vi "Get Classes to Inherit From.vi"(8 "error in (no error)":errorcluster, 11 "New Class Dialog In":refnum<class "New Class Dialog.lvclass">) -> (0 "error out":errorcluster, 3 "New Class Dialog Out":refnum<class "New Class Dialog.lvclass">)   [LabVIEW 2020, in "Process Generation.lvlib" / "New Class Dialog.lvclass"]
uses:
  New Class Dialog.lvclass
  Framework/Process/Process.lvclass
  Framework/Application/Application.lvclass
  C:/Users/anton/Documents/GitHub/Triarc-Framework/source/Framework/Process/Process.lvclass
  Framework/View/View.lvclass
  New Class Dialog.lvclass/New Class Dialog.ctl
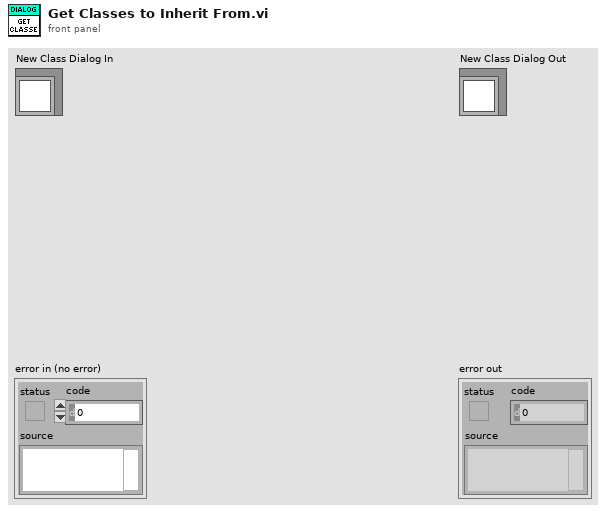
[diagram p1: front panel]
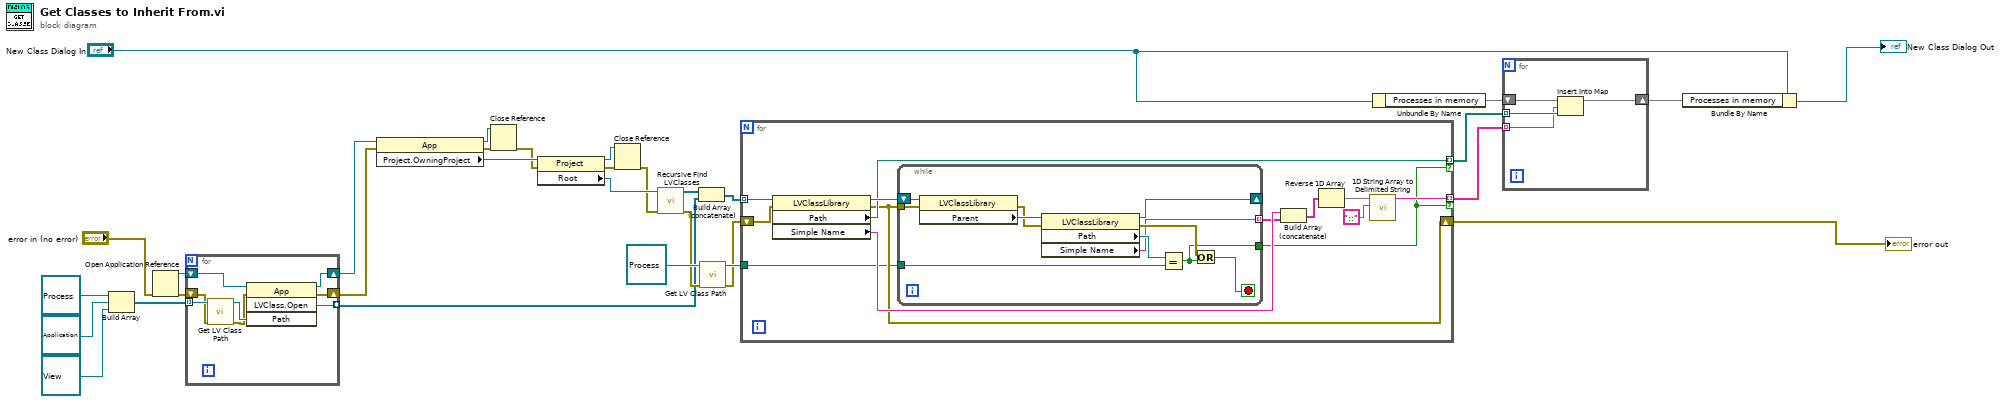
[diagram p0: block diagram]
diagram:
  n1 = Build Array(refnum<class "Process.lvclass"> refnum ("Process.lvclass"), refnum<class "Application.lvclass"> refnum ("Application.lvclass"), refnum<class "View.lvclass"> refnum ("View.lvclass")) -> (w8:refnum<class "Process.lvclass">[])
  n2 = Open Application Reference(8:"error in (no error)") -> (0:w5:errorcluster, 3:w4:refnum<vi>)  [unwired: 3 in]
  n3 = for {
    tunnel: w8 -> [w39] mode=indexing
    tunnel: [w37] -> w6 mode=indexing
    shift-right: [w35] -> w1
    shift-left: w4 -> [w34]
    shift-right: [w33] -> w2
    shift-left: w5 -> [w32]
    n4 = call <vilib>:"Get LV Class Path.vi"("error in (no error)"=w32, "object"=w39) -> ("error out"=w36:errorcluster, "class path"=w38:path)  [unwired: 8 in]
    n5 = invoke class="App" method="LVClass.Open"(reference=w34, error in=w36, "Path"=w38) -> (reference out=w35:refnum<vi>, error out=w33:errorcluster, "LVClass.Open"=w37:refnum<vi>)  [unwired: 1 in, 1 out]
  }
  n6 = property class="App"(reference=w1, error in=w2) -> (reference out=w12:refnum<vi>, error out=w14:errorcluster, "Project.OwningProject"=w15:refnum<vi>)
  n7 = Close Reference(reference=w12, error in (no error)=w14) -> (error out=w13:errorcluster)
  n8 = property class="Project"(reference=w15, error in=w13) -> (reference out=w21:refnum<vi>, error out=w20:errorcluster, "Root"=w19:refnum<vi>)
  n9 = Close Reference(reference=w21, error in (no error)=w20) -> (error out=w18:errorcluster)
  n10 = call "Recursive Find LVClasses.vi"("error in (no error)"=w18, "reference"=w19) -> ("error out"=w17:errorcluster, "Class References"=w16:refnum<vi>[])  [unwired: 8 in]
  n11 = Build Array (concatenate)(w16, w6) -> (w7:refnum<vi>[])
  n12 = call <vilib>:"Get LV Class Path.vi"("error in (no error)"=w17, "object"=refnum<class "Process.lvclass"> refnum ("Process.lvclass")) -> ("error out"=w22:errorcluster, "class path"=w24:path)  [unwired: 8 in]
  n13 = for {
    tunnel: w7 -> [w52] mode=indexing
    shift-right: [w41] -> w31
    shift-left: w22 -> [w50]
    tunnel: [w44] -> w28 mode=indexing if=w42
    tunnel: [w43] -> w27 mode=indexing if=w42
    tunnel: w24 -> [w40]
    n14 = property class="LVClassLibrary"(reference=w52, error in=w50) -> (reference out=w51:refnum<vi>, error out=w41:errorcluster, "Path"=w43:path, "Simple Name"=w46:string)
    n15 = while {
      tunnel: w41 -> [w59]
      tunnel: [w56] -> w45 mode=indexing
      tunnel: [w55] -> w42
      shift-right: [w54] -> _
      shift-left: w51 -> [w63]
      tunnel: w40 -> [w53]
      stop <- w57 stop-if-true
      n16 = property class="LVClassLibrary"(reference=w63, error in=w59) -> (error out=w60:errorcluster, "Parent"=w62:refnum<vi>)  [unwired: 1 out]
      n17 = property class="LVClassLibrary"(reference=w62, error in=w60) -> (reference out=w54:refnum<vi>, error out=w58:errorcluster, "Path"=w61:path, "Simple Name"=w56:string)
      n18 = Equal?(x=w61, y=w53) -> (x = y?=w55:bool)
      n19 = Or(x=w58, y=w55) -> (x .or. y?=w57:bool)
    }
    n20 = Build Array (concatenate)(w46, w45) -> (w49:string[])
    n21 = Reverse 1D Array(array=w49) -> (reversed array=w48:string[])
    n22 = call <vilib>:"1D String Array to Delimited String.vi"("delimiter"="::", "string array"=w48) -> ("delimited string"=w44:string)  [unwired: 9 in]
  }
  "error out" <- w31
  n23 = Unbundle By Name("New Class Dialog In") -> ("Processes in memory"=w26:map{string, path})
  n24 = for {
    shift-right: [w64] -> w25
    shift-left: w26 -> [w67]
    tunnel: w27 -> [w66] mode=indexing
    tunnel: w28 -> [w65] mode=indexing
    n25 = Insert Into Map(map in=w67, key=w65, value=w66) -> (map out=w64:map{string, path})  [unwired: 2 out]
  }
  n26 = Bundle By Name(cluster="New Class Dialog In", "Processes in memory"=w25) -> (→"New Class Dialog Out":refnum<class "New Class Dialog.lvclass">)
